vi "Create FPGA Addon.vi"(7 "Configuration (.dat)":path, 8 "error in (no error)":errorcluster, 9 "RIO Device (Use Config if Empty)":string, 10 "Name":string, 11 "Custom Devices Ref":refnum<k24>) -> (0 "error out":errorcluster, 3 "Custom Devices Ref":refnum<k24>)   [LabVIEW 2019, in "FPGA System Definition API.lvlib"]
uses:
  FPGA System Definition API.lvlib
  NationalInstruments.VeriStand.SystemDefinitionAPI
  Addon/Addon Shared/SubVIs/Constants.vi
  <vilib>/NI/NI VeriStand Advanced SysDef API/_SubVIs/SysDef.Property.Set.String.vi
  <vilib>/NI/NI VeriStand Custom Device Import and Export Tool/ImportExport.lvlib
  Addon/Addon Shared/FPGA Addon Shared.lvlib
  <vilib>/NI/NI VeriStand Advanced SysDef API/SysDef API/Advanced System Definition.lvlib
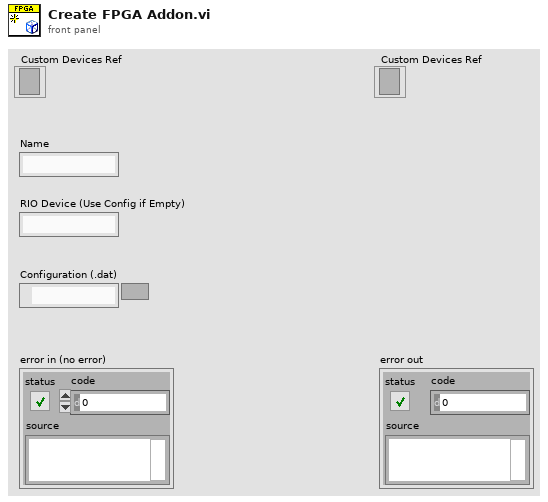
[diagram p1: front panel]
types:
  T1 = typedef "Custom Device API.lvlib/Custom Device Item Ref.ctl" = u64
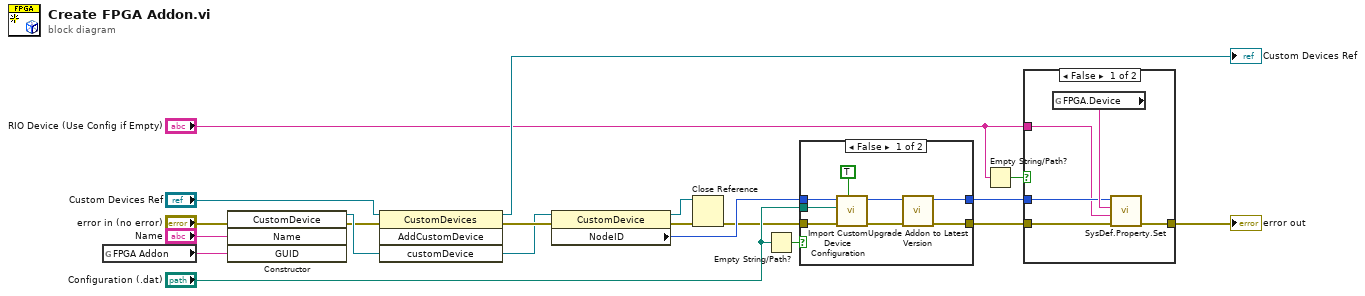
[diagram p0: block diagram]
diagram:
  n1 = global read "Constants.vi" "FPGA Addon"() -> (w14:string)
  n2 = constructor class="CustomDevice"(error in="error in (no error)", "Name"="Name", "GUID"=w14) -> (reference out=w10:refnum<k24>, error out=w9:errorcluster)  [unwired: 2 in, 3 out]
  n3 = invoke class="CustomDevices" method="AddCustomDevice"(reference="Custom Devices Ref", error in=w9, "customDevice"=w10) -> (reference out=→"Custom Devices Ref":refnum<k24>, error out=w19:errorcluster)  [unwired: 1 in, 2 out]
  n4 = property class="CustomDevice"(reference=w10, error in=w19) -> (reference out=w17:refnum<k24>, error out=w18:errorcluster, "NodeID"=w7:u64)
  n5 = Close Reference(reference=w17, error in (no error)=w18) -> (error out=w6:errorcluster)
  n6 = Empty String/Path?(string/path="Configuration (.dat)") -> (empty?=w15:bool)
  n7 = case shown="False" w15 {
    tunnel: [w20 w29] -> w4
    tunnel: w6 -> [w27 w29]
    tunnel: w7 -> [w26 w28]
    tunnel: "Configuration (.dat)" -> [w25 _]
    tunnel: [w21 w28] -> w1
    frame False {
      n8 = call <vilib>:"Import Custom Device Configuration.vi"("Overwrite Existing?"=TRUE, "error in (no error)"=w27, "Path"=w25, "NodeID"=w26) -> ("error out"=w23:errorcluster, "NodeID out"=w22:u64)  [unwired: 5 in, 1 out]
      n9 = call "Upgrade Addon to Latest Version.vi"("error in (no error)"=w23, "Device Item Ref in in"=w22) -> ("error out"=w20:errorcluster, "Device Item Ref out"=w21:T1)  [unwired: 8 in]
    }
    frame True {
    }
  }
  n10 = Empty String/Path?(string/path="RIO Device (Use Config if Empty)") -> (empty?=w8:bool)
  n11 = case shown="False" w8 {
    tunnel: w4 -> [w34 w35]
    tunnel: [w33 w35] -> w3
    tunnel: w1 -> [w31 _]
    tunnel: "RIO Device (Use Config if Empty)" -> [w30 _]
    frame False {
      n12 = global read "Constants.vi" "FPGA.Device"() -> (w32:string)
      n13 = call-poly <vilib>:"SysDef.Property.Set.vi"("error in (no error)"=w34, "Value"=w30, "Property Name"=w32, "nodeID"=w31) -> ("error out"=w33:errorcluster)  [unwired: 6 in, 1 out]
    }
    frame True {
    }
  }
  "error out" <- w3
